vi "Call Python.vi"(8 "error in (no error)":errorcluster) -> (0 "error out":errorcluster, 3 "String":string)   [LabVIEW 2019]
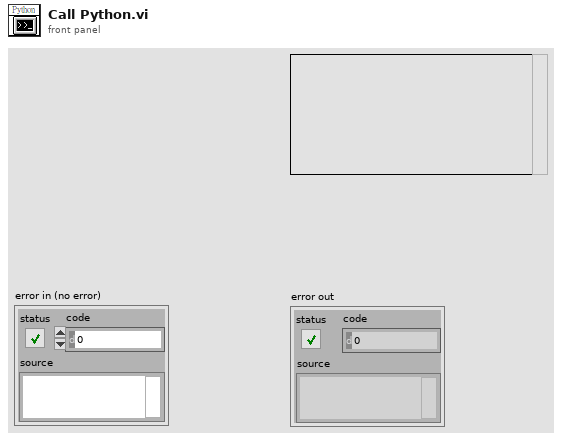
[diagram p1: front panel]
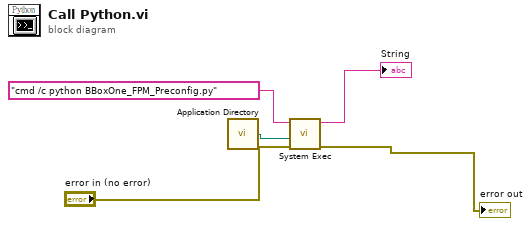
[diagram p0: block diagram]
diagram:
  n1 = call <vilib>:"Application Directory.vi"() -> ("Application Directory"=w4:path)
  n2 = call <vilib>:"System Exec.vi"("error in (no error)"="error in (no error)", "working directory"=w4, "command line"="cmd /c python BBoxOne_FPM_Preconfig.py") -> ("error out"=→"error out":errorcluster, "standard output"=→"String":string)  [unwired: 5 in, 2 out]
